vi "FileConversions.vi"() -> ()   [LabVIEW 2022 SP3]
panel:
  in  "Convert":bool
  in  "Conversion":T1(ring)
  in  "Destination Path":path caption="selected path"
  in  "Source Path":path caption="selected path"
  out "Array":path[](array[path])
  # "File Conversion Assistant"
  # "1. select conversion"
  # "2. Select parent folder\n      of existing files"
  # "3. Select where you want\n    the new files to go"
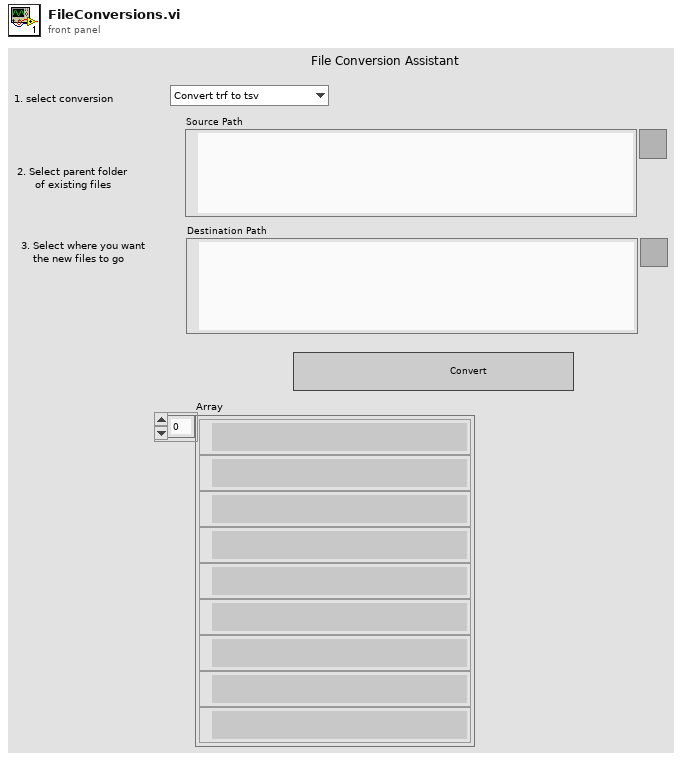
[diagram p1: front panel]
types:
  T1 = enum16{"Convert trf to tsv", "Convert trf to csv", "Convert trf to wav", "Convert wfm to tsv", "Convert wfm to csv", "Convert wfm to wav"}
  T2 = cluster{"Start freq":dbl, "Hz resolution":dbl, dbl[]}
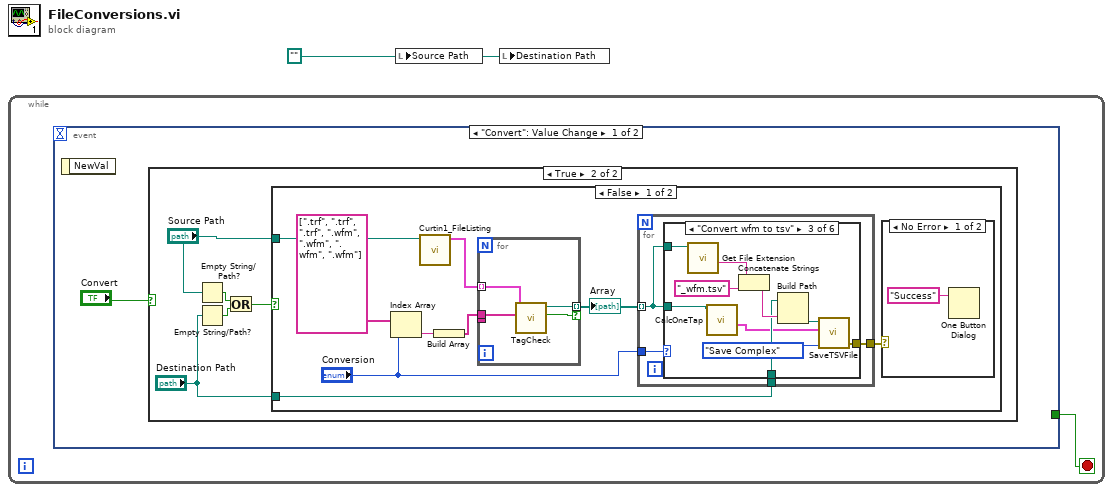
[diagram p0: block diagram]
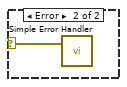
[diagram p3: hidden frame]
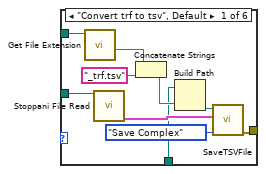
[diagram p4: hidden frame]
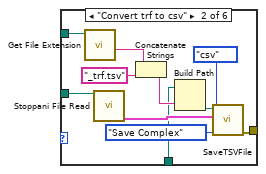
[diagram p5: hidden frame]
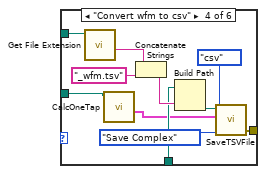
[diagram p6: hidden frame]
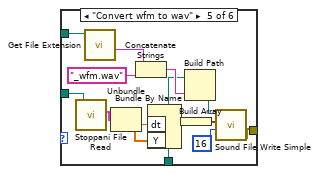
[diagram p7: hidden frame]
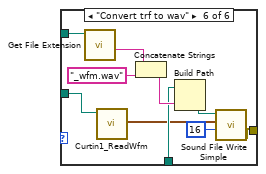
[diagram p8: hidden frame]
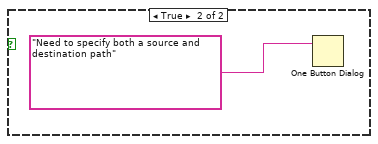
[diagram p9: hidden frame]
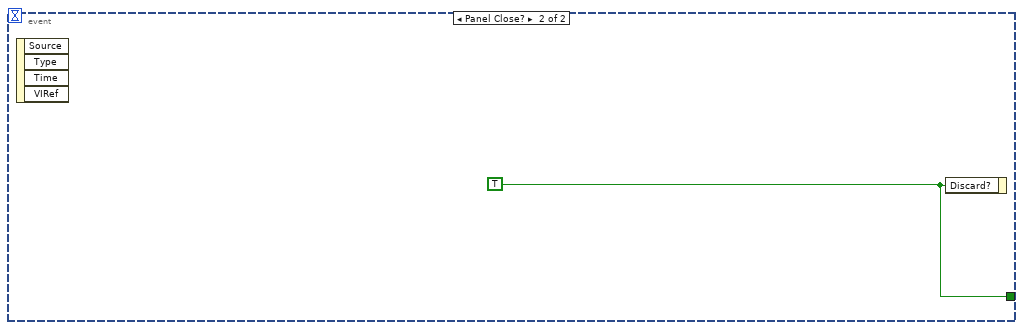
[diagram p10: hidden frame]
diagram:
  w1 = path ""
  n1 = while {
    stop <- w2 stop-if-true
    n2 = event shown="[0] \"Convert\": Value Change" {
      selector: _ -> [_ _]
      dyn-events: _ -> [_ _]
      timeout: _ -> [_ _]
      tunnel: [_ w95] -> w2
      event "Convert": Value Change {
        n3 = event-data() -> ()  [unwired: 1 in, 1 out]
        n4 = case shown="True" "Convert" {
          frame False {
          }
          frame True {
            n5 = Empty String/Path?(string/path="Source Path") -> (empty?=w6:bool)
            n6 = Empty String/Path?(string/path="Destination Path") -> (empty?=w7:bool)
            n7 = Or(x=w6, y=w7) -> (x .or. y?=w5:bool)
            n8 = case shown="False" w5 {
              tunnel: "Source Path" -> [w16 _]
              tunnel: "Destination Path" -> [w10 _]
              frame False {
                n9 = Index Array(array=string[] [".trf", ".trf", ".trf", ".wfm", ".wfm", ".wfm", ".wfm"], index="Conversion") -> (element=w14:string)
                n10 = call "Curtin1_FileListing.vi"("Folder Path"=w16) -> ("Array"=w17:cluster{"Folder Path":path, "tags":string[]}[])  [unwired: 10 in]
                n11 = Build Array(w14) -> (w13:string[])
                n12 = for {
                  tunnel: [w90] -> _
                  tunnel: [w93] -> w12 mode=indexing if=w92
                  tunnel: w17 -> [w91] mode=indexing
                  tunnel: w13 -> [w90]
                  n13 = call "TagCheck.vi"("Tags"=w90, 11:w91) -> ("Good?"=w92:bool, "Path out"=w93:path)  [unwired: 8 in]
                }
                "Array" <- w12
                n14 = for {
                  tunnel: w12 -> [w22] mode=indexing
                  tunnel: "Conversion" -> [w23]
                  tunnel: w10 -> [w21]
                  tunnel: [w20] -> w9
                  n15 = case shown="\"Convert wfm to tsv\"" w23 {
                    tunnel: w22 -> [w33 w44 w48 w59 w71 w83]
                    tunnel: w22 -> [w28 w39 w51 w62 w76 w86]
                    tunnel: w21 -> [w26 w37 w49 w60 w75 w85]
                    tunnel: [w24 w35 w45 w56 w72 w80] -> w20
                    frame "Convert trf to tsv", Default {
                      n16 = call <vilib>:"Get File Extension.vi"("file"=w28) -> ("filename without extension"=w31:string)  [unwired: 6 in, 4 out]
                      n17 = call "Stoppani File Read.vi"("String in"=w33) -> ("Complex FRF"=w32:cluster{"t0":dbl, "dt":dbl, "Y":cdb[]})  [unwired: 2 in, 3 out]
                      n18 = Concatenate Strings(w31, "_trf.tsv" ("string")) -> (w29:string)
                      n19 = Build Path(base path=w26, name or relative path=w29) -> (appended path=w27:path)
                      n20 = call "SaveTSVFile.vi"("Task"=enum16{"Save Magnitude", "Save Complex"}."Save Complex", "FRF"=w32, "Path"=w27) -> ("error out"=w24:errorcluster)  [unwired: 8 in]
                    }
                    frame "Convert trf to csv" {
                      n21 = call <vilib>:"Get File Extension.vi"("file"=w39) -> ("filename without extension"=w42:string)  [unwired: 6 in, 4 out]
                      n22 = call "Stoppani File Read.vi"("String in"=w44) -> ("Complex FRF"=w43:cluster{"t0":dbl, "dt":dbl, "Y":cdb[]})  [unwired: 2 in, 3 out]
                      n23 = Concatenate Strings(w42, "_trf.tsv" ("string")) -> (w40:string)
                      n24 = Build Path(base path=w37, name or relative path=w40) -> (appended path=w38:path)
                      n25 = call "SaveTSVFile.vi"("Task"=enum16{"Save Magnitude", "Save Complex"}."Save Complex", "type"=enum16{"tsv", "csv"}."csv", "FRF"=w43, "Path"=w38) -> ("error out"=w35:errorcluster)  [unwired: 7 in]
                    }
                    frame "Convert wfm to tsv" {
                      n26 = call <vilib>:"Get File Extension.vi"("file"=w51) -> ("filename without extension"=w54:string)  [unwired: 6 in, 4 out]
                      n27 = call "CalcOneTap.vi"("wavform file"=w48) -> ("Complex FRF"=w47:cluster{dbl, "df":dbl, cdb[]})  [unwired: 7 in, 3 out]
                      n28 = Concatenate Strings(w54, "_wfm.tsv" ("string")) -> (w52:string)
                      n29 = Build Path(base path=w49, name or relative path=w52) -> (appended path=w50:path)
                      n30 = call "SaveTSVFile.vi"("Task"=enum16{"Save Magnitude", "Save Complex"}."Save Complex", "FRF"=w47, "Path"=w50) -> ("error out"=w45:errorcluster)  [unwired: 8 in]
                    }
                    frame "Convert wfm to csv" {
                      n31 = call <vilib>:"Get File Extension.vi"("file"=w62) -> ("filename without extension"=w65:string)  [unwired: 6 in, 4 out]
                      n32 = call "CalcOneTap.vi"("wavform file"=w59) -> ("Complex FRF"=w58:cluster{dbl, "df":dbl, cdb[]})  [unwired: 7 in, 3 out]
                      n33 = Concatenate Strings(w65, "_wfm.tsv" ("string")) -> (w63:string)
                      n34 = Build Path(base path=w60, name or relative path=w63) -> (appended path=w61:path)
                      n35 = call "SaveTSVFile.vi"("Task"=enum16{"Save Magnitude", "Save Complex"}."Save Complex", "type"=enum16{"tsv", "csv"}."csv", "FRF"=w58, "Path"=w61) -> ("error out"=w56:errorcluster)  [unwired: 7 in]
                    }
                    frame "Convert wfm to wav" {
                      n36 = call "Stoppani File Read.vi"("String in"=w71) -> ("Waveform Graph"=w70:T2)  [unwired: 2 in, 3 out]
                      n37 = call <vilib>:"Get File Extension.vi"("file"=w76) -> ("filename without extension"=w79:string)  [unwired: 6 in, 4 out]
                      n38 = Unbundle(w70) -> ("Hz resolution"=w69:dbl, w68:dbl[])  [unwired: 1 out]
                      n39 = Concatenate Strings(w79, "_wfm.wav" ("string")) -> (w77:string)
                      n40 = Bundle By Name("dt"=w69, "Y"=w68) -> (w67:waveform(dbl))  [unwired: 1 in]
                      n41 = Build Array(w67) -> (w66:waveform(dbl)[])
                      n42 = Build Path(base path=w75, name or relative path=w77) -> (appended path=w74:path)
                      n43 = call <vilib>:"Sound File Write Simple.vi"("bits per sample"=16, "data"=w66, "path"=w74) -> ("error out"=w72:errorcluster)  [unwired: 7 in, 1 out]
                    }
                    frame "Convert trf to wav" {
                      n44 = call <vilib>:"Get File Extension.vi"("file"=w86) -> ("filename without extension"=w89:string)  [unwired: 6 in, 4 out]
                      n45 = call "Curtin1_ReadWfm.vi"("appended path"=w83) -> ("all waveforms in record"=w84:waveform(dbl)[])  [unwired: 9 in, 1 out]
                      n46 = Concatenate Strings(w89, "_wfm.wav" ("string")) -> (w87:string)
                      n47 = Build Path(base path=w85, name or relative path=w87) -> (appended path=w82:path)
                      n48 = call <vilib>:"Sound File Write Simple.vi"("bits per sample"=16, "data"=w84, "path"=w82) -> ("error out"=w80:errorcluster)  [unwired: 7 in, 1 out]
                    }
                  }
                }
                n49 = case shown="No Error" w9 {
                  selector: w9 -> [_ w19]
                  frame No Error {
                    n50 = One Button Dialog(message="Success") -> ()  [unwired: 1 in, 1 out]
                  }
                  frame Error {
                    n51 = call <vilib>:"Simple Error Handler.vi"("error in (no error)"=w19) -> ()  [unwired: 4 in, 5 out]
                  }
                }
              }
              frame True {
                n52 = One Button Dialog(message="Need to specify both a source and destination path") -> ()  [unwired: 1 in, 1 out]
              }
            }
          }
        }
      }
      event Panel Close? {
        w95 = TRUE ("Discard?")
        n53 = event-data() -> ()  [unwired: 1 in, 4 out]
        n54 = event-data("Discard?"=w95) -> ()  [unwired: 1 in, 1 out]
      }
    }
  }
  n55 = local write "Source Path"(w1) -> ()
  n56 = local write "Destination Path"(w1) -> ()
